vi "Read Cell String.vi"(0 "Report Ref In":T1, 1 "Row Index":i32, 2 "Column Index":i32, 3 "error in (no error)":errorcluster) -> (4 "Value":string, 5 "Report Ref Out":T1, 6 "error out":errorcluster)   [LabVIEW 2026, in "XCel Report Engine.lvlib"]
doc: "Reads the value of a cell from the active worksheet and returns it as a string.\n\nThe cell can be specified using an Excel A1 address or zero-based row and column coordinates, depending on the implemented connector interface. Coordinate (0, 0) corresponds to cell A1.\n\nAn empty or missing cell returns an empty string. Boolean values are returned as TRUE or FALSE, and numeric values use their invariant-culture representation.\n\nIf the cell contains a formula, this VI returns an error. XCelReportEngine does not evaluate formulas or return cached formula results; any required calculation must be performed by the LabVIEW application."
uses:
  XCel Report Engine.lvlib
  Controls/Report Ref.ctl
  C:/Users/weird/Desktop/XCelReportEngine/LV/DotNet/XCelReportEngine.dll
  DotNet/XCelReportEngine.dll
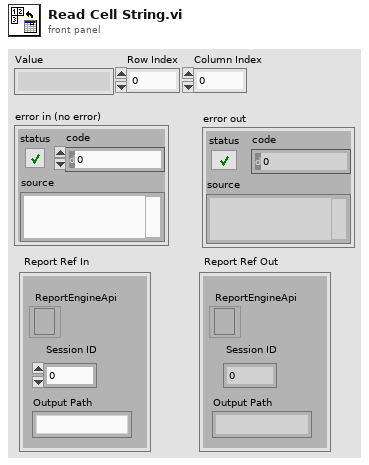
[diagram p1: front panel]
types:
  T1 = typedef "XCel Report Engine.lvlib/Report Ref.ctl" = cluster{"Session ID":i32, "Output Path":string, "ReportEngineApi":refnum<k24>}
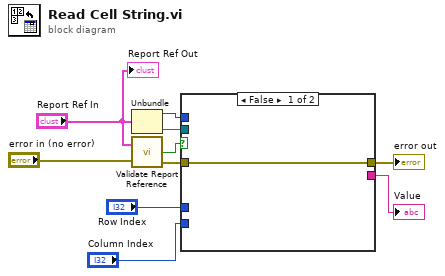
[diagram p0: block diagram]
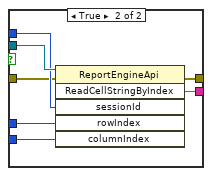
[diagram p2: hidden frame]
diagram:
  n1 = Unbundle("Report Ref In") -> ("Session ID"=w8:i32, "ReportEngineApi"=w10:refnum<k24>)  [unwired: 1 out]
  n2 = call "Validate Report Reference.vi"("Report Ref In"="Report Ref In", "error in (no error)"="error in (no error)") -> ("Valid"=w1:bool, "error out"=w2:errorcluster)  [unwired: 1 out]
  n3 = case shown="False" w1 {
    tunnel: w10 -> [_ w18]
    tunnel: [w11 w17] -> w9
    tunnel: w8 -> [_ w16]
    tunnel: "Row Index" -> [_ w15]
    tunnel: "Column Index" -> [_ w14]
    tunnel: [_ w13] -> w5
    tunnel: w2 -> [w11 w12]
    frame False {
    }
    frame True {
      n4 = invoke class="ReportEngineApi" method="ReadCellStringByIndex"(reference=w18, error in=w12, "sessionId"=w16, "rowIndex"=w15, "columnIndex"=w14) -> (error out=w17:errorcluster, "ReadCellStringByIndex"=w13:string)  [unwired: 1 in, 4 out]
    }
  }
  "error out" <- w9
  "Value" <- w5
  "Report Ref Out" <- "Report Ref In"
